vi "Fluidic Process.vi"(8 "error in":errorcluster) -> (0 "error out":errorcluster)   [LabVIEW 2019, in "Fluidic Process.lvlib"]
uses:
  Fluidic Process.lvlib
  User Event/Controls/UE Abort Action.ctl
  SubVI/Fluidic Para.ctl
  SubVI/Fluidic Data.ctl
  IO/sbRIO9623/SubVI/IO Control.ctl
  <vilib>/Utility/error.llb/Error Cluster From Error Code.vi
  <vilib>/ErrorRing/Error Ring.xnode
  Queues/Queues.lvlib
  Syringe Pump/NE-500/NE-500.lvlib
  Selection Valve/IDEX/IDEX.lvlib
  IO/sbRIO9623/sbRIO9623.lvlib
  LED/LED.lvlib
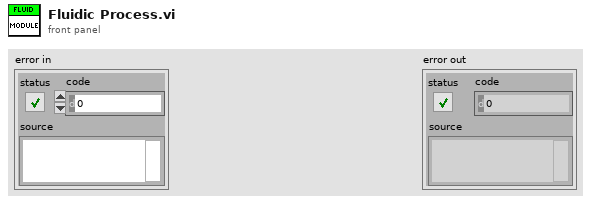
[diagram p1: front panel]
types:
  T1 = typedef "Fluidic Process.lvlib/Fluidic Para.ctl" = cluster{"Read Force Sensor":i32, "Read Regulator":i32, "Read Force Sensor?":bool, "Read Regulator?":bool, "Read Syringe Pump":i32, "Read Syringe Pump?":bool}
  T2 = typedef "Fluidic Process.lvlib/Fluidic Data.ctl" = cluster{"Step":i32, "Duration Time(s)":i32, "Syringe Pump Control":cluster{"Withdraw Rate (ul/min)":dbl, "Infuse Rate (ul/min)":dbl, "Direction":enum16{"Infuse", "Withdraw"}, "Syringe Diameter(mm)":dbl, "Syringe Pump Switch":bool}, "Selection Valve":enum16{"No Action", "Position 1", "Position 2", "Position 3", "Position 4", "Position 5", "Position 6"}, "Buffer Pinch Valve":cluster{"Buffer Load L":bool, "Buffer Load R":bool, "Buffer Chip L":bool, "Buffer Chip R":bool, "Sorting Waste":bool, "Filter Waste":bool, "Reagent Waste":bool, "Buffer Waste":bool, "Wash/Buffer Tank":bool}, "Blood Pinch Valve":cluster{"Load S1":bool, "Load S2":bool, "Blood in":bool}, "Regulator":cluster{"BL2 (V)":fxp<+,16,3>, "BL1 (V)":fxp<+,16,3>, "BR1 (V)":fxp<+,16,3>, "BR2 (V)":fxp<+,16,3>}, "Fast Valve":cluster{"Fast Valve 1":bool, "Fast Valve 2":bool}, "Air Valve":bool, "Blood Tube Latch1":bool, "Buffer Pump":bool, "Blood Sensor":cluster{"Calibrate Sensor 1":bool, "Calibrate Sensor 2":bool}, "Mirror Change":enum16{"Camera Side", "SiPM Side"}}
  T3 = cluster{"Fluidic Para":T1, "Total Process":i32, "Current Process":i32, "Tick Count":u32, "Duration(s)":dbl, "Fluidic Process":T2[], "Current Fluidic Process":T2, "Total Duration(s)":dbl, "Duration(s) Array":dbl[]}
  T4 = typedef "UE Abort Action.ctl" = enum16{"Create", "Get", "Destroy"}
  T5 = cluster{"Wdr Rate(UM)":dbl, "Inf Rate(UM)":dbl, "Dir":enum16{"Infuse", "Withdraw"}, "Dia(mm)":dbl}
  T6 = typedef "sbRIO9623.lvlib/IO Control.ctl" = cluster{"Regulator":cluster{"BL2 (V)":fxp<+,16,3>, "BL1 (V)":fxp<+,16,3>, "BR1 (V)":fxp<+,16,3>, "BR2 (V)":fxp<+,16,3>}, "Buffer Pinch Valve":cluster{"Buffer Load L":bool, "Buffer Load R":bool, "Buffer Chip L":bool, "Buffer Chip R":bool, "Sorting Waste":bool, "Filter Waste":bool, "Reagent Waste":bool, "Buffer Waste":bool, "Wash/Buffer Tank":bool}, "Blood Pinch Valve":cluster{"Load S1":bool, "Load S2":bool, "Blood in":bool}, "Fast Valve":cluster{"Fast Valve 1":bool, "Fast Valve 2":bool}, "Blood Sensor":cluster{"Calibrate Sensor 1":bool, "Calibrate Sensor 2":bool}, "Air Pressure":cluster{"Air Compressor":bool, "Air Compressor Manual":bool}, "Blood Tube Latch1":bool, "Air Valve":bool, "Buffer Pump":bool, "Mirror Change":enum16{"Camera Side", "SiPM Side"}}
  T7 = typedef "Fluidic Process.lvlib/SEQ Data.ctl" = cluster{"Fluidic Process Done?":bool, "Current Process":i32, "Remaining Time":dbl, "Total Process":i32, "Air Sealing":bool, "Force Condition":bool}
  T8 = typedef "LED.lvlib/SEQ Data.ctl" = cluster{"Initialize Sucess?":bool, "BL2 Regulator":dbl, "BL1 Regulator":dbl, "Blood Sensor 1":dbl, "Blood Sensor 2":dbl, "Air Pressure Sensor":dbl, "Force Snesor 1":u32, "Force Snesor 2":u32, "VI Refnum":refnum<vi>}
  T9 = cluster{"Withdraw Rate (ul/min)":dbl, "Infuse Rate (ul/min)":dbl, "Direction":enum16{"Infuse", "Withdraw"}, "Syringe Diameter(mm)":dbl, "Syringe Pump Switch":bool}
  T10 = enum16{"No Action", "Position 1", "Position 2", "Position 3", "Position 4", "Position 5", "Position 6"}
  T11 = typedef "NE-500.lvlib/SEQ Data.ctl" = cluster{"Status":string, "Initialize Done?":bool, "VI Refnum":refnum<vi>}
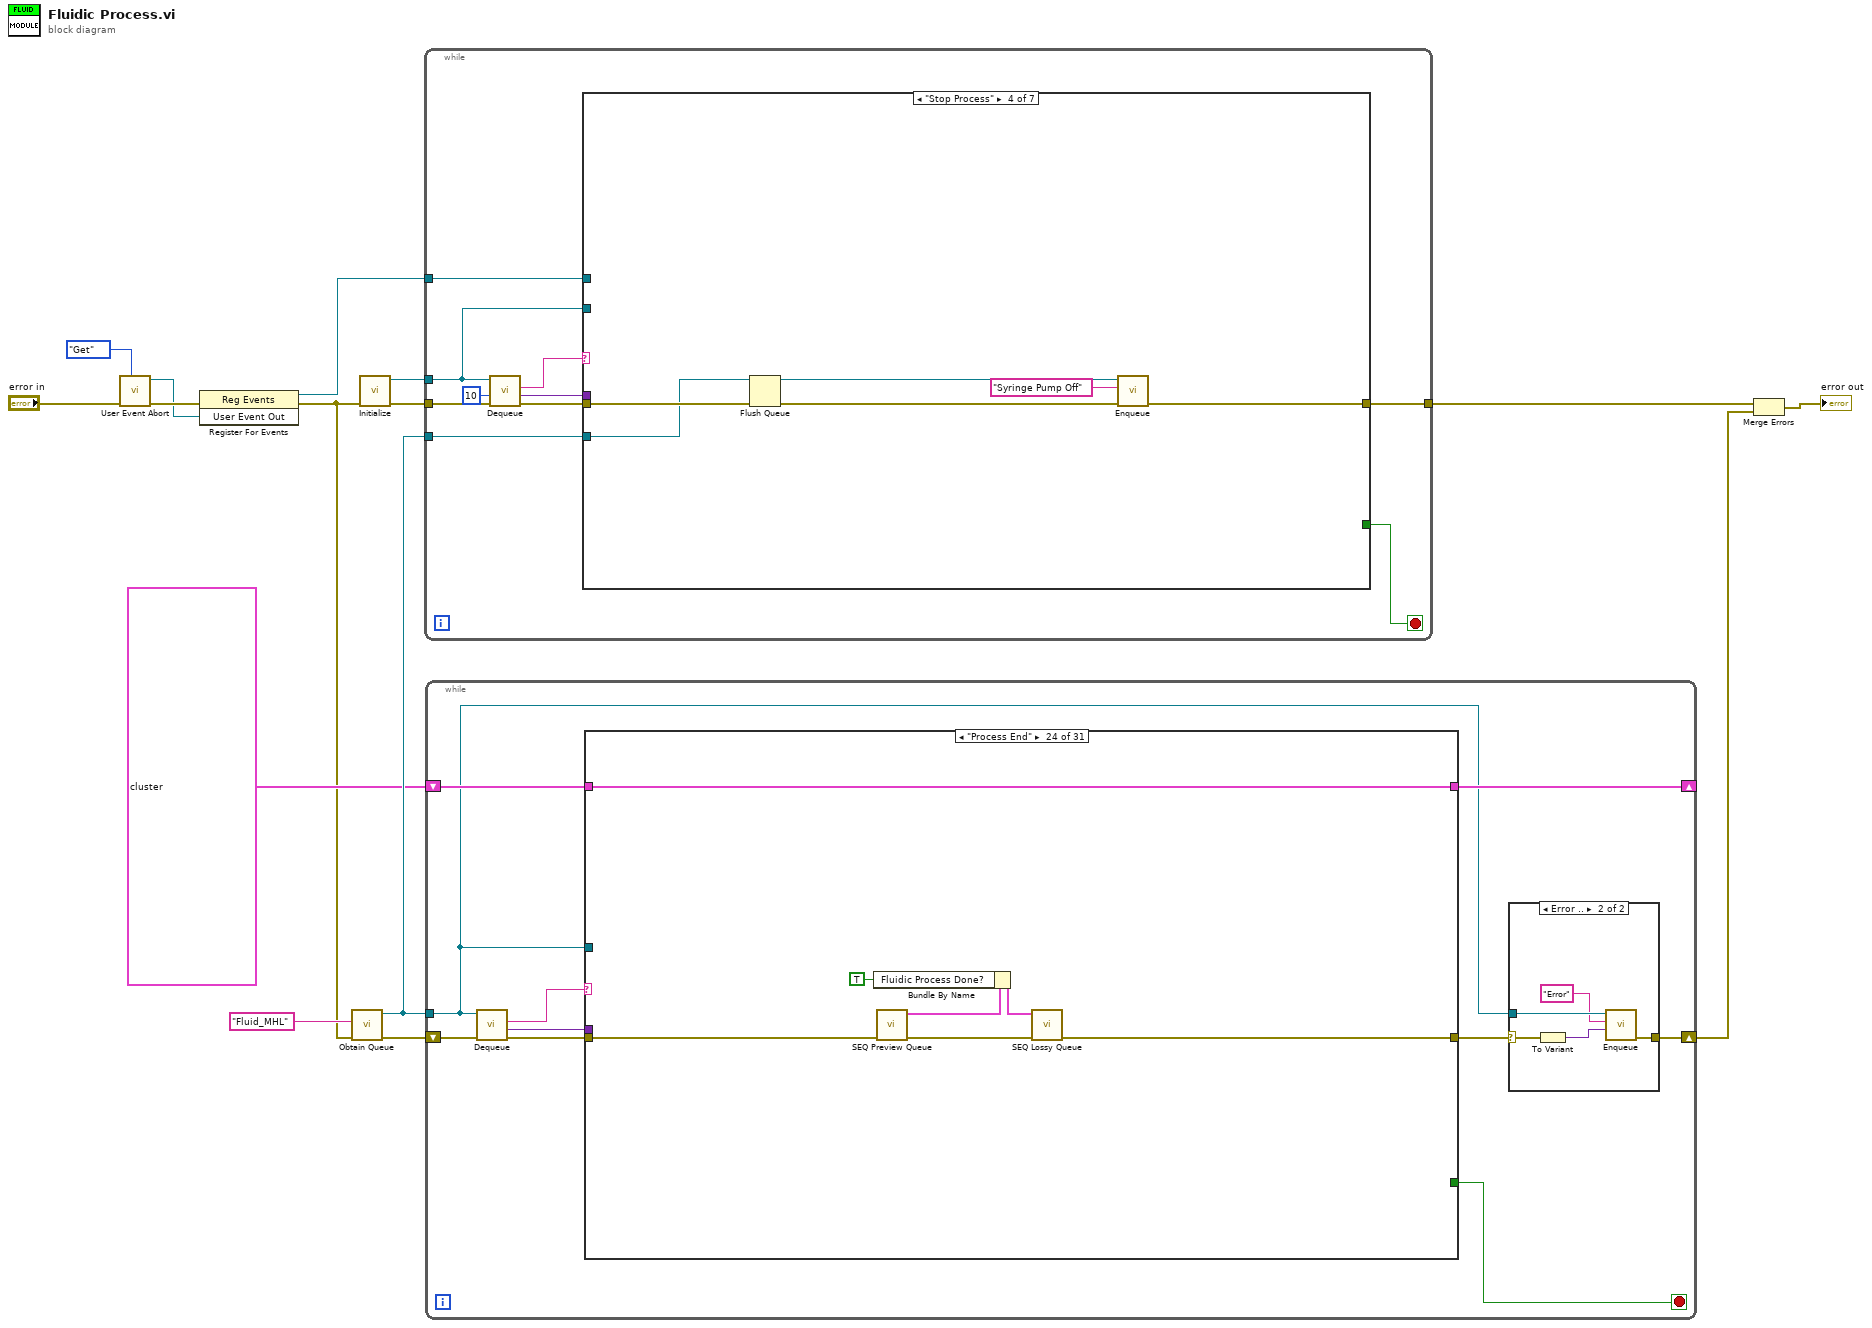
[diagram p0: block diagram]
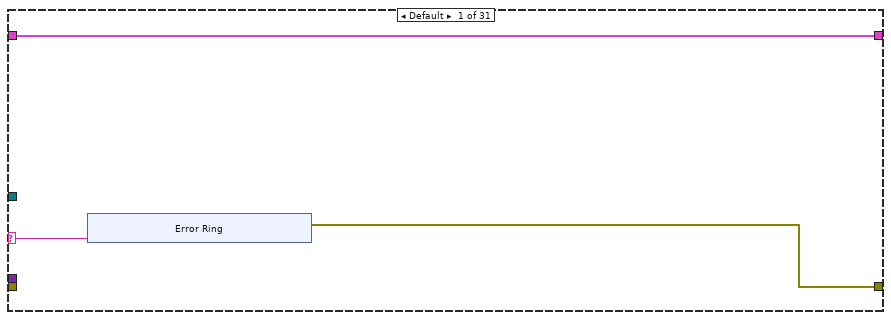
[diagram p2: hidden frame]
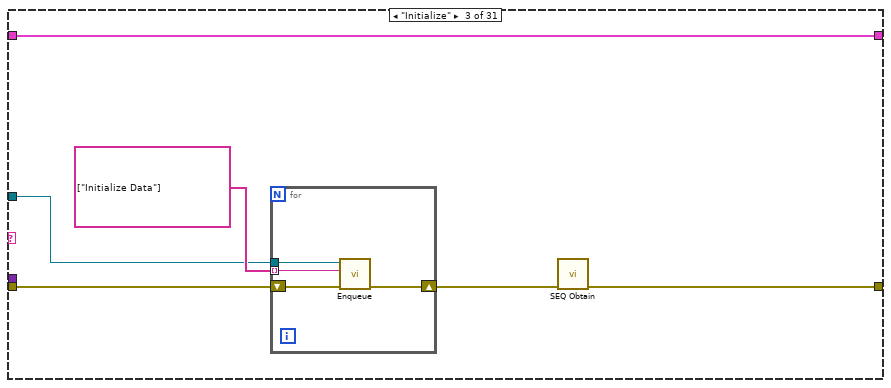
[diagram p4: hidden frame]
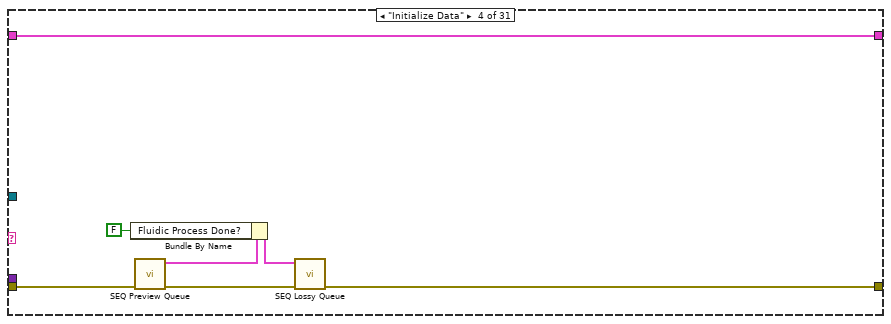
[diagram p5: hidden frame]
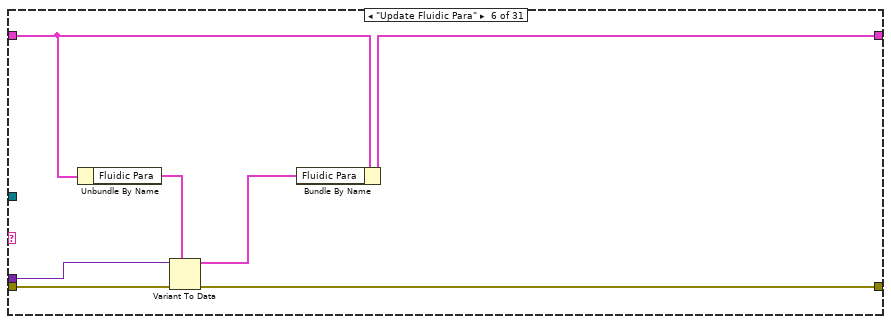
[diagram p7: hidden frame]
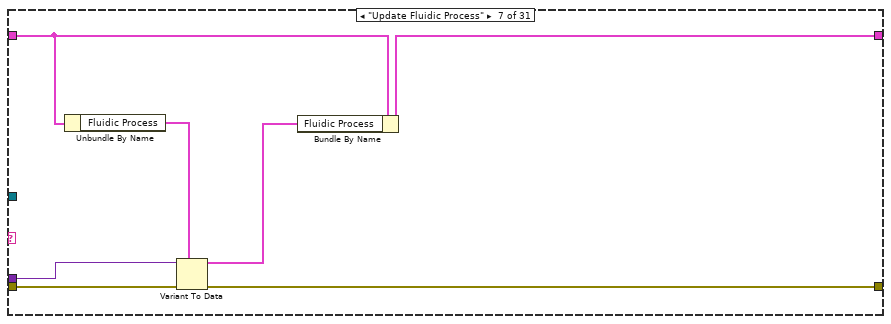
[diagram p8: hidden frame]
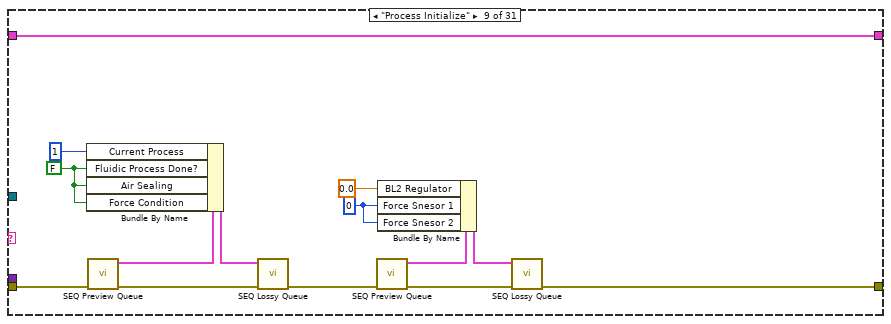
[diagram p10: hidden frame]
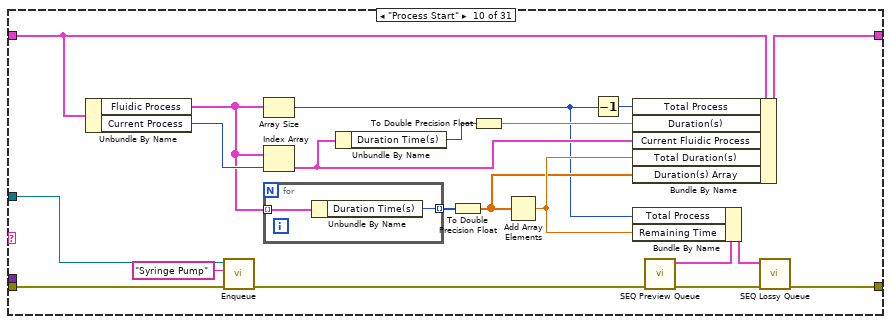
[diagram p11: hidden frame]
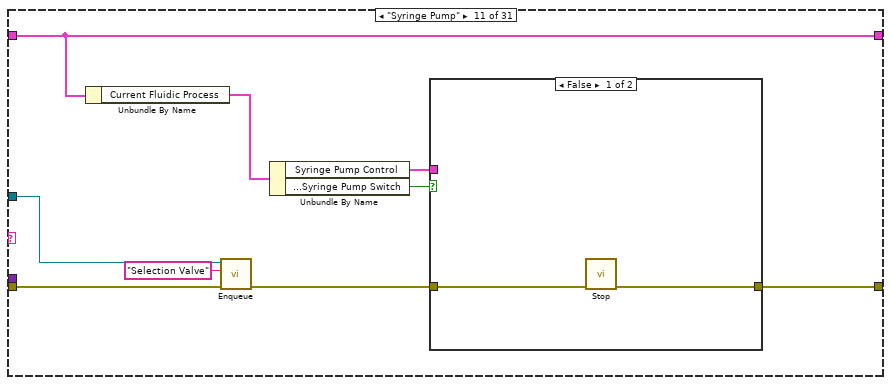
[diagram p12: hidden frame]
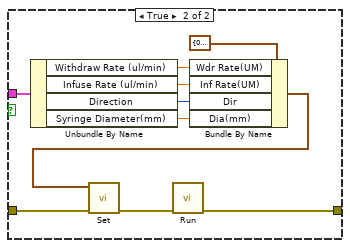
[diagram p13: hidden frame]
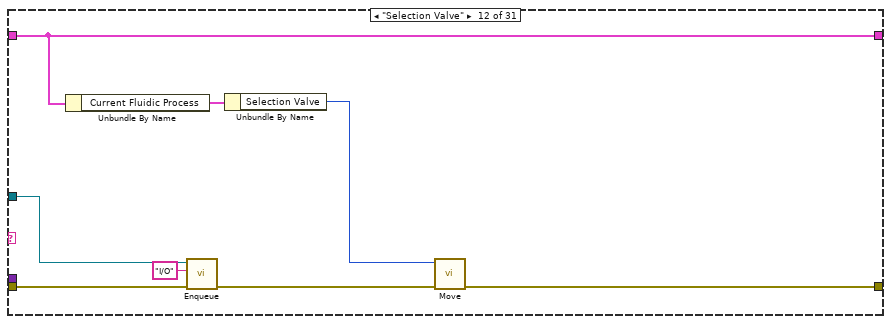
[diagram p14: hidden frame]
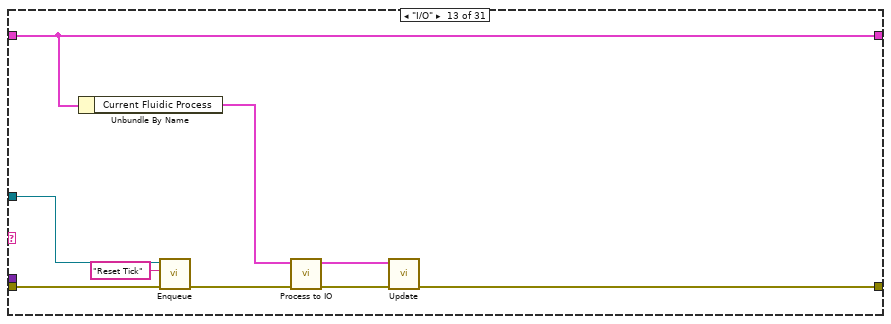
[diagram p15: hidden frame]
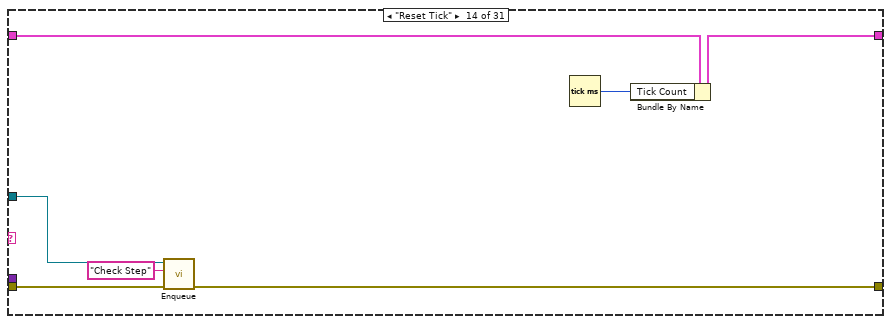
[diagram p16: hidden frame]
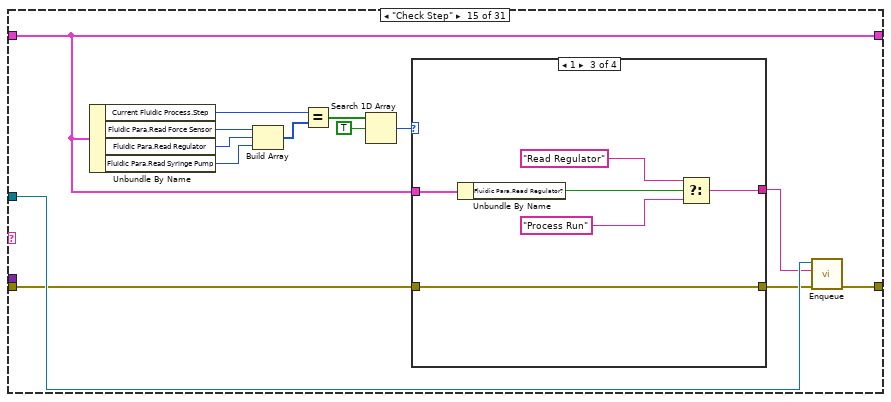
[diagram p17: hidden frame]
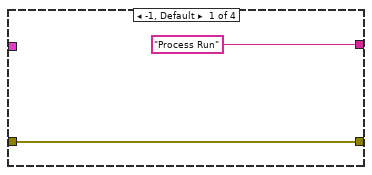
[diagram p18: hidden frame]
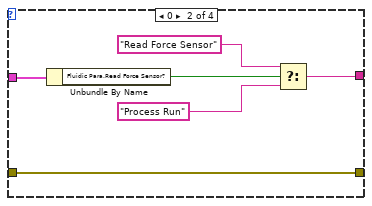
[diagram p19: hidden frame]
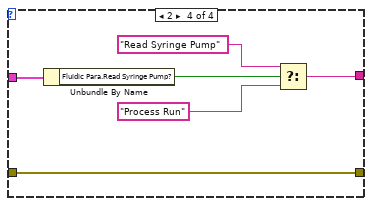
[diagram p20: hidden frame]
diagram:
  n1 = call "User Event Abort.vi"("Action"=UE_Abort_Action."Get", "Error In"="error in") -> ("Error Out"=w13:errorcluster, "User Event Out"=w12:refnum<user-event>)  [unwired: 8 in]
  n2 = register-events(error in=w13, w12) -> (reference out=w11:refnum<event-registration>, error out=w3:errorcluster)  [unwired: 1 in]
  n3 = call "Obtain Queue.vi"("Error In"=w3, "Queue Name"="Fluid_MHL") -> ("Error Out"=w9:errorcluster, "queue out"=w5:refnum<queue>)  [unwired: 8 in]
  n4 = call "Initialize.vi"("Error In"=w3) -> ("Error Out"=w2:errorcluster, "Queue out"=w1:refnum<queue>)  [unwired: 9 in]
  n5 = while {
    tunnel: w2 -> [w25]
    tunnel: w1 -> [w20]
    tunnel: [w19] -> w8
    tunnel: w11 -> [w18]
    tunnel: w5 -> [w16]
    stop <- w17 stop-if-true
    n6 = call "Dequeue.vi"("Error In"=w25, "timeout in ms (-1)"=10, "Queue in"=w20) -> ("Error Out"=w24:errorcluster, "Data"=w22:variant, "State"=w23:string)  [unwired: 5 in, 1 out]
    n7 = case shown="\"Stop Process\"" w23 {
      selector: w23 -> [w26 _ _ _ _ _ _]
      tunnel: w24 -> [w29 w33 w50 w60 w66 w70 w78]
      tunnel: w22 -> [_ _ w49 _ w63 _ _]
      tunnel: w20 -> [_ _ _ _ _ _ _]
      tunnel: [w29 w32 w43 w61 w65 w69 w77] -> w19
      tunnel: w18 -> [_ _ _ _ _ _ w76]
      tunnel: [_ _ _ _ _ TRUE _] -> w17
      tunnel: w16 -> [_ w31 w45 w58 w64 w68 _]
      frame "Typo", Default {
        n8 = Concatenate Strings("Typo: " ("string"), w26) -> (w28:string)
        n9 = One Button Dialog(message=w28) -> ()  [unwired: 1 in, 1 out]
      }
      frame "Initialize" {
        n10 = for {
          tunnel: w31 -> [w35]
          shift-right: [w36] -> w32
          shift-left: w33 -> [w37]
          tunnel: string[] ["Initialize"] -> [w34] mode=indexing
          n11 = call "Enqueue.vi"("Error In"=w37, "State"=w34, "Queue in"=w35) -> ("Error Out"=w36:errorcluster)  [unwired: 7 in, 1 out]
        }
      }
      frame "Run Process" {
        w40 = variant
        n12 = Variant To Data(error in=w50, type=string[][] [] ("Fluidic Process in"), Variant=w49) -> (data=w46:string[][], error out=w47:errorcluster)
        n13 = call "Prcoess Converter.vi"("error in"=w47, "Fluidic Process in"=w46) -> ("error out"=w44:errorcluster, "Fluidic Process out"=w42:T2[])  [unwired: 8 in]
        n14 = To Variant(anything=w42) -> (Variant=w41:variant)
        n15 = Build Array(w40, w41, w40) -> (w38:variant[])
        n16 = for {
          tunnel: w45 -> [w55]
          shift-right: [w53] -> w43
          shift-left: w44 -> [w54]
          tunnel: string[] ["Process Initialize", "Update Fluidic Process", "Process Start"] -> [w52] mode=indexing
          tunnel: w38 -> [w51] mode=indexing
          n17 = call "Enqueue.vi"("Error In"=w54, "Data"=w51, "State"=w52, "Queue in"=w55) -> ("Error Out"=w53:errorcluster)  [unwired: 6 in, 1 out]
        }
      }
      frame "Stop Process" {
        n18 = Flush Queue(queue=w58, error in (no error)=w60) -> (queue out=w57:refnum<queue>, error out=w59:errorcluster)  [unwired: 1 out]
        n19 = call "Enqueue.vi"("Error In"=w59, "State"="Syringe Pump Off", "Queue in"=w57) -> ("Error Out"=w61:errorcluster)  [unwired: 7 in, 1 out]
      }
      frame "Update Fluidic Para" {
        n20 = call "Enqueue.vi"("Error In"=w66, "Data"=w63, "State"="Update Fluidic Para", "Queue in"=w64) -> ("Error Out"=w65:errorcluster)  [unwired: 6 in, 1 out]
      }
      frame "Close" {
        n21 = for {
          tunnel: w68 -> [w73]
          shift-right: [w74] -> w69
          shift-left: w70 -> [w75]
          tunnel: string[] ["Close"] -> [w72] mode=indexing
          n22 = call "Enqueue.vi"("Error In"=w75, "State"=w72, "Queue in"=w73) -> ("Error Out"=w74:errorcluster)  [unwired: 7 in, 1 out]
        }
      }
      frame "Idle" {
        n23 = event shown="[1] <User Event Out>: User Event" {
          selector: w76 -> [_ w84]
          dyn-events: _ -> [_ _]
          timeout: 10 -> [_ _]
          tunnel: w78 -> [w80 w82]
          tunnel: [w80 w83] -> w77
          event Timeout {
            n24 = event-data() -> ()  [unwired: 1 in, 3 out]
          }
          event User Event {
            n25 = event-data() -> ()  [unwired: 1 in, 4 out]
            n26 = call "Close.vi"("Error In"=w82) -> ("Error Out"=w81:errorcluster)  [unwired: 10 in]
            n27 = Unregister For Events(event registration refnum=w84, error in=w81) -> (error out=w83:errorcluster)
          }
        }
      }
    }
  }
  n28 = while {
    tunnel: w5 -> [w86]
    shift-right: [w89] -> _
    shift-left: T3 {"Fluidic Para"={"Read Force Sensor"=0, "Read Regulator"=0, "Read Force Sensor?"=FALSE, "Read Regulator?"=FALSE, "Read Syringe Pump"=0, "Read Syringe Pump?"=FALSE}, "Total Process"=0, "Current Process"=0, "Tick Count"=0, "Duration(s)"=0.0, "Fluidic Process"=[], "Current Fluidic Process"={"Step"=0, "Duration Time(s)"=0, "Syringe Pump Control"={"Withdraw Rate (ul/min)"=0.0, "Infuse Rate (ul/min)"=0.0, "Direction"=enum."Infuse", "Syringe Diameter(mm)"=0.0, "Syringe Pump Switch"=FALSE}, "Selection Valve"=enum."No Action", "Buffer Pinch Valve"={"Buffer Load L"=FALSE, "Buffer Load R"=FALSE, "Buffer Chip L"=FALSE, "Buffer Chip R"=FALSE, "Sorting Waste"=FALSE, "Filter Waste"=FALSE, "Reagent Waste"=FALSE, "Buffer Waste"=FALSE, "Wash/Buffer Tank"=FALSE}, "Blood Pinch Valve"={"Load S1"=FALSE, "Load S2"=FALSE, "Blood in"=FALSE}, "Regulator"={"BL2 (V)"=0.0, "BL1 (V)"=0.0, "BR1 (V)"=0.0, "BR2 (V)"=0.0}, "Fast Valve"={"Fast Valve 1"=FALSE, "Fast Valve 2"=FALSE}, "Air Valve"=FALSE, "Blood Tube Latch1"=FALSE, "Buffer Pump"=FALSE, "Blood Sensor"={"Calibrate Sensor 1"=FALSE, "Calibrate Sensor 2"=FALSE}, "Mirror Change"=enum."Camera Side"}, "Total Duration(s)"=0.0, "Duration(s) Array"=[]} -> [w90]
    shift-right: [w88] -> w6
    shift-left: w9 -> [w94]
    stop <- w85 stop-if-true
    n29 = call "Dequeue.vi"("Error In"=w94, "Queue in"=w86) -> ("Error Out"=w91:errorcluster, "Data"=w92:variant, "State"=w93:string)  [unwired: 6 in, 1 out]
    n30 = case shown="\"Process End\"" w93 {
      selector: w93 -> [w96 _ _ _ _ _ _ _ _ _ _ _ _ _ _ _ _ _ _ _ _ _ _ _ _ _ _ _ _ _ _]
      tunnel: w86 -> [_ _ w110 _ _ _ _ _ _ w170 w185 w205 w214 w220 w235 w260 w266 w271 w297 w334 w369 w404 w417 _ w455 w464 _ _ _ w479 w489]
      tunnel: w92 -> [_ _ _ _ _ w131 w138 _ _ _ _ _ _ _ _ _ _ _ _ _ _ _ _ _ _ _ _ w471 _ _ _]
      tunnel: w91 -> [_ w105 w111 w122 w125 w132 w139 w140 w155 w173 w186 w206 w215 w221 w225 w261 w267 w272 w298 w324 w359 w379 w419 w449 w456 w465 w468 w472 w476 w480 w490]
      tunnel: w90 -> [w97 w106 w109 w123 w124 w130 w137 w141 w142 w175 w184 w204 w213 w222 w226 w262 w268 w273 w279 w315 w348 w393 w426 w450 w457 w466 w467 w469 w475 w477 w488]
      tunnel: [w97 w106 w109 w123 w124 w128 w135 w141 w142 w174 w184 w204 w213 w217 w226 w262 w268 w273 w279 w315 w348 w393 w425 w450 w457 w466 w467 w469 w475 w477 w488] -> w89
      tunnel: [w95 w105 w107 w120 w125 w126 w133 w140 w148 w162 w180 w200 w208 w218 w236 w258 w264 w269 w284 w311 w353 w389 w413 w447 w451 w461 w468 errorcluster {"status"=FALSE, "code"=0, "source"=""} ("Error Out") w476 w478 w486] -> w87
      tunnel: [_ _ _ _ _ _ _ _ _ _ _ _ _ _ _ _ _ _ _ _ _ _ _ _ _ _ _ _ _ _ TRUE] -> w85
      frame Default {
        n31 = xnode "Error Ring"("parameter 0"=w96) -> ("error out"=w95:errorcluster)
      }
      frame "------Initialize------" {
      }
      frame "Initialize" {
        n32 = for {
          tunnel: w110 -> [w114]
          shift-right: [w115] -> w108
          shift-left: w111 -> [w116]
          tunnel: string[] ["Initialize Data"] -> [w113] mode=indexing
          n33 = call "Enqueue.vi"("Error In"=w116, "State"=w113, "Queue in"=w114) -> ("Error Out"=w115:errorcluster)  [unwired: 7 in, 1 out]
        }
        n34 = call "SEQ Obtain.vi"("error in"=w108) -> ("error out"=w107:errorcluster)  [unwired: 9 in, 1 out]
      }
      frame "Initialize Data" {
        n35 = call "SEQ Preview Queue.vi"("error in"=w122) -> ("error out"=w121:errorcluster, "SEQ Data"=w119:T7)  [unwired: 9 in]
        n36 = Bundle By Name(cluster=w119, "Fluidic Process Done?"=FALSE) -> (w118:T7)
        n37 = call "SEQ Lossy Queue.vi"("error in"=w121, "SEQ Data"=w118) -> ("error out"=w120:errorcluster)  [unwired: 9 in]
      }
      frame "------Functions------" {
      }
      frame "Update Fluidic Para" {
        n38 = Unbundle By Name(w130) -> ("Fluidic Para"=w129:T1)
        n39 = Variant To Data(error in=w132, type=w129, Variant=w131) -> (data=w127:T1, error out=w126:errorcluster)
        n40 = Bundle By Name(cluster=w130, "Fluidic Para"=w127) -> (w128:T3)
      }
      frame "Update Fluidic Process" {
        n41 = Unbundle By Name(w137) -> ("Fluidic Process"=w136:T2[])
        n42 = Variant To Data(error in=w139, type=w136, Variant=w138) -> (data=w134:T2[], error out=w133:errorcluster)
        n43 = Bundle By Name(cluster=w137, "Fluidic Process"=w134) -> (w135:T3)
      }
      frame "------Process------" {
      }
      frame "Process Initialize" {
        w144 = u32 0 ("Force Snesor 1")
        w143 = FALSE ("Fluidic Process Done?")
        n44 = call "SEQ Preview Queue.vi"("error in"=w155) -> ("error out"=w154:errorcluster, "SEQ Data"=w153:T7)  [unwired: 9 in]
        n45 = Bundle By Name(cluster=w153, "Current Process"=1, "Fluidic Process Done?"=w143, "Air Sealing"=w143, "Force Condition"=w143) -> (w152:T7)
        n46 = call "SEQ Lossy Queue.vi"("error in"=w154, "SEQ Data"=w152) -> ("error out"=w150:errorcluster)  [unwired: 9 in]
        n47 = call "SEQ Preview Queue.vi"("error in"=w150) -> ("error out"=w149:errorcluster, "SEQ Data"=w147:T8)  [unwired: 9 in]
        n48 = Bundle By Name(cluster=w147, "BL2 Regulator"=0.0, "Force Snesor 1"=w144, "Force Snesor 2"=w144) -> (w146:T8)
        n49 = call "SEQ Lossy Queue.vi"("error in"=w149, "SEQ Data"=w146) -> ("error out"=w148:errorcluster)  [unwired: 9 in]
      }
      frame "Process Start" {
        n50 = Unbundle By Name(w175) -> ("Fluidic Process"=w165:T2[], "Current Process"=w171:i32)
        n51 = call "Enqueue.vi"("Error In"=w173, "State"="Syringe Pump", "Queue in"=w170) -> ("Error Out"=w164:errorcluster)  [unwired: 7 in, 1 out]
        n52 = Array Size(array=w165) -> (size(s)=w156:i32)
        n53 = Index Array(array=w165, index=w171) -> (element=w168:T2)
        n54 = for {
          tunnel: w165 -> [w177] mode=indexing
          tunnel: [w176] -> w159 mode=indexing
          n55 = Unbundle By Name(w177) -> ("Duration Time(s)"=w176:i32)
        }
        n56 = Unbundle By Name(w168) -> ("Duration Time(s)"=w167:i32)
        n57 = To Double Precision Float(number=w159) -> (double precision float=w157:dbl[])
        n58 = To Double Precision Float(number=w167) -> (double precision float=w166:dbl)
        n59 = Add Array Elements(numeric array=w157) -> (sum=w158:dbl)
        n60 = Decrement(x=w156) -> (x-1=w172:i32)
        n61 = Bundle By Name(cluster=w175, "Total Process"=w172, "Duration(s)"=w166, "Current Fluidic Process"=w168, "Total Duration(s)"=w158, "Duration(s) Array"=w157) -> (w174:T3)
        n62 = call "SEQ Preview Queue.vi"("error in"=w164) -> ("error out"=w163:errorcluster, "SEQ Data"=w161:T7)  [unwired: 9 in]
        n63 = Bundle By Name(cluster=w161, "Total Process"=w156, "Remaining Time"=w158) -> (w160:T7)
        n64 = call "SEQ Lossy Queue.vi"("error in"=w163, "SEQ Data"=w160) -> ("error out"=w162:errorcluster)  [unwired: 9 in]
      }
      frame "Syringe Pump" {
        n65 = Unbundle By Name(w184) -> ("Current Fluidic Process"=w183:T2)
        n66 = call "Enqueue.vi"("Error In"=w186, "State"="Selection Valve", "Queue in"=w185) -> ("Error Out"=w181:errorcluster)  [unwired: 7 in, 1 out]
        n67 = Unbundle By Name(w183) -> ("Syringe Pump Control"=w179:T9, "Syringe Pump Control.Syringe Pump Switch"=w182:bool)
        n68 = case shown="False" w182 {
          tunnel: w181 -> [w188 w198]
          tunnel: [w187 w189] -> w180
          tunnel: w179 -> [_ w196]
          frame False {
            n69 = call "Stop.vi"("Error In"=w188) -> ("Error Out"=w187:errorcluster)  [unwired: 10 in]
          }
          frame True {
            n70 = Unbundle By Name(w196) -> ("Withdraw Rate (ul/min)"=w194:dbl, "Infuse Rate (ul/min)"=w193:dbl, "Direction"=w192:enum16{"Infuse", "Withdraw"}, "Syringe Diameter(mm)"=w191:dbl)
            n71 = Bundle By Name(cluster=T5 {"Wdr Rate(UM)"=0.0, "Inf Rate(UM)"=0.0, "Dir"=enum."Infuse", "Dia(mm)"=0.0} ("Setting"), "Wdr Rate(UM)"=w194, "Inf Rate(UM)"=w193, "Dir"=w192, "Dia(mm)"=w191) -> (w190:T5)
            n72 = call "Set.vi"("Error In"=w198, "Setting"=w190) -> ("Error Out"=w197:errorcluster)  [unwired: 9 in]
            n73 = call "Run.vi"("Error In"=w197) -> ("Error Out"=w189:errorcluster)  [unwired: 10 in]
          }
        }
      }
      frame "Selection Valve" {
        n74 = Unbundle By Name(w204) -> ("Current Fluidic Process"=w203:T2)
        n75 = call "Enqueue.vi"("Error In"=w206, "State"="I/O", "Queue in"=w205) -> ("Error Out"=w201:errorcluster)  [unwired: 7 in, 1 out]
        n76 = Unbundle By Name(w203) -> ("Selection Valve"=w202:T10)
        n77 = call "Move.vi"("Error In"=w201, "Position"=w202) -> ("Error Out"=w200:errorcluster)  [unwired: 9 in]
      }
      frame "I/O" {
        n78 = Unbundle By Name(w213) -> ("Current Fluidic Process"=w212:T2)
        n79 = call "Enqueue.vi"("Error In"=w215, "State"="Reset Tick", "Queue in"=w214) -> ("Error Out"=w211:errorcluster)  [unwired: 7 in, 1 out]
        n80 = call "Process to IO.vi"("error in"=w211, "Process in"=w212) -> ("error out"=w210:errorcluster, "Process out"=w209:T6)  [unwired: 8 in]
        n81 = call "Update.vi"("Error In"=w210, "I/O Control"=w209) -> ("Error Out"=w208:errorcluster)  [unwired: 9 in]
      }
      frame "Reset Tick" {
        n82 = call "Enqueue.vi"("Error In"=w221, "State"="Check Step", "Queue in"=w220) -> ("Error Out"=w218:errorcluster)  [unwired: 7 in, 1 out]
        n83 = Tick Count (ms)() -> (millisecond timer value=w216:u32)
        n84 = Bundle By Name(cluster=w222, "Tick Count"=w216) -> (w217:T3)
      }
      frame "Check Step" {
        n85 = Unbundle By Name(w226) -> ("Current Fluidic Process.Step"=w231:i32, "Fluidic Para.Read Force Sensor"=w234:i32, "Fluidic Para.Read Regulator"=w233:i32, "Fluidic Para.Read Syringe Pump"=w232:i32)
        n86 = Build Array(w234, w233, w232) -> (w230:i32[])
        n87 = Equal?(x=w231, y=w230) -> (x = y?=w229:bool[])
        n88 = Search 1D Array(1D array=w229, element=TRUE) -> (index of element=w227:i32)  [unwired: 1 in]
        n89 = case shown="1" w227 {
          tunnel: w226 -> [_ w243 w249 w255]
          tunnel: w225 -> [w238 w244 w250 w256]
          tunnel: [w238 w244 w250 w256] -> w224
          tunnel: ["Process Run" w239 w245 w251] -> w223
          frame -1, Default {
          }
          frame 0 {
            n90 = Unbundle By Name(w243) -> ("Fluidic Para.Read Force Sensor?"=w240:bool)
            n91 = Select(t="Read Force Sensor", s=w240, f="Process Run") -> (s? t:f=w239:string)
          }
          frame 1 {
            n92 = Unbundle By Name(w249) -> ("Fluidic Para.Read Regulator?"=w246:bool)
            n93 = Select(t="Read Regulator", s=w246, f="Process Run") -> (s? t:f=w245:string)
          }
          frame 2 {
            n94 = Unbundle By Name(w255) -> ("Fluidic Para.Read Syringe Pump?"=w252:bool)
            n95 = Select(t="Read Syringe Pump", s=w252, f="Process Run") -> (s? t:f=w251:string)
          }
        }
        n96 = call "Enqueue.vi"("Error In"=w224, "State"=w223, "Queue in"=w235) -> ("Error Out"=w236:errorcluster)  [unwired: 7 in, 1 out]
      }
      frame "Read Force Sensor" {
        n97 = call "Enqueue.vi"("Error In"=w261, "State"="Process Run_Force Sensor", "Queue in"=w260) -> ("Error Out"=w259:errorcluster)  [unwired: 7 in, 1 out]
        n98 = call "Read Force Sensor.vi"("Error In"=w259) -> ("Error Out"=w258:errorcluster)  [unwired: 10 in]
      }
      frame "Read Regulator" {
        n99 = call "Enqueue.vi"("Error In"=w267, "State"="Process Run_Regulator", "Queue in"=w266) -> ("Error Out"=w265:errorcluster)  [unwired: 7 in, 1 out]
        n100 = call "Read BL2 Regulator.vi"("Error In"=w265) -> ("Error Out"=w264:errorcluster)  [unwired: 10 in]
      }
      frame "Read Syringe Pump" {
        n101 = call "Enqueue.vi"("Error In"=w272, "State"="Process Run_Syringe Pump", "Queue in"=w271) -> ("Error Out"=w269:errorcluster)  [unwired: 7 in, 1 out]
      }
      frame "Process Run" {
        n102 = Unbundle By Name(w279) -> ("Total Duration(s)"=w281:dbl, "Tick Count"=w296:u32, "Duration(s)"=w291:dbl)
        n103 = Tick Count (ms)() -> (millisecond timer value=w295:u32)
        n104 = Subtract(x=w295, y=w296) -> (x-y=w294:u32)
        n105 = To Double Precision Float(number=w294) -> (double precision float=w293:dbl)
        n106 = Divide(x=w293, y=1000.0) -> (x/y=w280:dbl)
        n107 = Wait (ms)(milliseconds to wait=u32 100) -> ()  [unwired: 1 out]
        n108 = Greater Or Equal?(x=w280, y=w291) -> (x >= y?=w290:bool)
        n109 = Subtract(x=w281, y=w280) -> (x-y=w274:dbl)
        n110 = Select(t="Process Next", s=w290, f="Process Run") -> (s? t:f=w287:string)
        n111 = Less?(x=w274, y=0.0) -> (x < y?=w276:bool)
        n112 = Select(t=0.0, s=w276, f=w274) -> (s? t:f=w277:dbl)
        n113 = call "Enqueue.vi"("Error In"=w298, "State"=w287, "Queue in"=w297) -> ("Error Out"=w286:errorcluster)  [unwired: 7 in, 1 out]
        n114 = call "SEQ Preview Queue.vi"("error in"=w286) -> ("error out"=w285:errorcluster, "SEQ Data"=w283:T7)  [unwired: 9 in]
        n115 = Bundle By Name(cluster=w283, "Remaining Time"=w277) -> (w282:T7)
        n116 = call "SEQ Lossy Queue.vi"("error in"=w285, "SEQ Data"=w282) -> ("error out"=w284:errorcluster)  [unwired: 9 in]
      }
      frame "Process Run_Force Sensor" {
        w319 = u32 220 ("y")
        n117 = Unbundle By Name(w315) -> ("Total Duration(s)"=w314:dbl, "Tick Count"=w333:u32, "Duration(s)"=w328:dbl)
        n118 = call "SEQ Preview Queue.vi"("error in"=w324) -> ("error out"=w323:errorcluster, "SEQ Data"=w322:T8)  [unwired: 9 in]
        n119 = Unbundle By Name(w322) -> ("Force Snesor 1"=w321:u32, "Force Snesor 2"=w320:u32)
        n120 = Tick Count (ms)() -> (millisecond timer value=w332:u32)
        n121 = Subtract(x=w332, y=w333) -> (x-y=w331:u32)
        n122 = To Double Precision Float(number=w331) -> (double precision float=w330:dbl)
        n123 = Greater Or Equal?(x=w321, y=w319) -> (x >= y?=w318:bool)
        n124 = Greater Or Equal?(x=w320, y=w319) -> (x >= y?=w317:bool)
        n125 = Divide(x=w330, y=1000.0) -> (x/y=w313:dbl)
        n126 = Greater Or Equal?(x=w313, y=w328) -> (x >= y?=w316:bool)
        n127 = And(x=w318, y=w317) -> (x .and. y?=w300:bool)
        n128 = Wait (ms)(milliseconds to wait=u32 100) -> ()  [unwired: 1 out]
        n129 = Or(x=w316, y=w300) -> (x .or. y?=w301:bool)
        n130 = Subtract(x=w314, y=w313) -> (x-y=w305:dbl)
        n131 = Select(t="Process Next", s=w301, f="Process Run_Force Sensor") -> (s? t:f=w325:string)
        n132 = Less?(x=w305, y=0.0) -> (x < y?=w307:bool)
        n133 = call "Enqueue.vi"("Error In"=w323, "State"=w325, "Queue in"=w334) -> ("Error Out"=w303:errorcluster)  [unwired: 7 in, 1 out]
        n134 = Select(t=0.0, s=w307, f=w305) -> (s? t:f=w304:dbl)
        n135 = case shown="True" w301 {
          tunnel: w303 -> [w336 w338]
          tunnel: [w336 w337] -> w302
          frame False {
          }
          frame True {
            n136 = call "Stop Read.vi"("Error In"=w338) -> ("Error Out"=w337:errorcluster)  [unwired: 10 in]
          }
        }
        n137 = call "SEQ Preview Queue.vi"("error in"=w302) -> ("error out"=w312:errorcluster, "SEQ Data"=w310:T7)  [unwired: 9 in]
        n138 = Bundle By Name(cluster=w310, "Remaining Time"=w304, "Force Condition"=w300) -> (w309:T7)
        n139 = call "SEQ Lossy Queue.vi"("error in"=w312, "SEQ Data"=w309) -> ("error out"=w311:errorcluster)  [unwired: 9 in]
      }
      frame "Process Run_Regulator" {
        n140 = Unbundle By Name(w348) -> ("Total Duration(s)"=w350:dbl, "Tick Count"=w368:u32, "Duration(s)"=w363:dbl)
        n141 = call "SEQ Preview Queue.vi"("error in"=w359) -> ("error out"=w358:errorcluster, "SEQ Data"=w357:T8)  [unwired: 9 in]
        n142 = Unbundle By Name(w357) -> ("BL2 Regulator"=w356:dbl)
        n143 = Tick Count (ms)() -> (millisecond timer value=w367:u32)
        n144 = Subtract(x=w367, y=w368) -> (x-y=w366:u32)
        n145 = To Double Precision Float(number=w366) -> (double precision float=w365:dbl)
        n146 = Greater?(x=w356, y=4.5) -> (0:w340:bool)
        n147 = Divide(x=w365, y=1000.0) -> (x/y=w349:dbl)
        n148 = Subtract(x=w350, y=w349) -> (x-y=w344:dbl)
        n149 = Greater Or Equal?(x=w349, y=w363) -> (x >= y?=w339:bool)
        n150 = Wait (ms)(milliseconds to wait=u32 100) -> ()  [unwired: 1 out]
        n151 = Select(t="Process Next", s=w339, f="Process Run_Regulator") -> (s? t:f=w360:string)
        n152 = Less?(x=w344, y=0.0) -> (x < y?=w346:bool)
        n153 = call "Enqueue.vi"("Error In"=w358, "State"=w360, "Queue in"=w369) -> ("Error Out"=w342:errorcluster)  [unwired: 7 in, 1 out]
        n154 = Select(t=0.0, s=w346, f=w344) -> (s? t:f=w343:dbl)
        n155 = case shown="False" w339 {
          tunnel: w342 -> [w371 w373]
          tunnel: [w371 w372] -> w341
          frame False {
          }
          frame True {
            n156 = call "Stop Read.vi"("Error In"=w373) -> ("Error Out"=w372:errorcluster)  [unwired: 10 in]
          }
        }
        n157 = call "SEQ Preview Queue.vi"("error in"=w341) -> ("error out"=w354:errorcluster, "SEQ Data"=w352:T7)  [unwired: 9 in]
        n158 = Bundle By Name(cluster=w352, "Remaining Time"=w343, "Air Sealing"=w340) -> (w351:T7)
        n159 = call "SEQ Lossy Queue.vi"("error in"=w354, "SEQ Data"=w351) -> ("error out"=w353:errorcluster)  [unwired: 9 in]
      }
      frame "Process Run_Syringe Pump" {
        n160 = Unbundle By Name(w393) -> ("Total Duration(s)"=w392:dbl, "Tick Count"=w403:u32, "Duration(s)"=w398:dbl)
        n161 = call "SEQ Preview Queue.vi"("error in"=w379) -> ("error out"=w378:errorcluster, "SEQ Data"=w377:T11)  [unwired: 9 in]
        n162 = Unbundle By Name(w377) -> ("Status"=w376:string)
        n163 = Tick Count (ms)() -> (millisecond timer value=w402:u32)
        n164 = Subtract(x=w402, y=w403) -> (x-y=w401:u32)
        n165 = Equal?(x=w376, y="P") -> (x = y?=w374:bool)
        n166 = To Double Precision Float(number=w401) -> (double precision float=w400:dbl)
        n167 = Divide(x=w400, y=1000.0) -> (x/y=w391:dbl)
        n168 = Greater Or Equal?(x=w391, y=w398) -> (x >= y?=w394:bool)
        n169 = Wait (ms)(milliseconds to wait=u32 100) -> ()  [unwired: 1 out]
        n170 = Or(x=w394, y=w374) -> (x .or. y?=w380:bool)
        n171 = Subtract(x=w392, y=w391) -> (x-y=w383:dbl)
        n172 = Select(t="Process Next", s=w380, f="Process Run_Syringe Pump") -> (s? t:f=w395:string)
        n173 = Less?(x=w383, y=0.0) -> (x < y?=w385:bool)
        n174 = call "Enqueue.vi"("Error In"=w378, "State"=w395, "Queue in"=w404) -> ("Error Out"=w381:errorcluster)  [unwired: 7 in, 1 out]
        n175 = Select(t=0.0, s=w385, f=w383) -> (s? t:f=w382:dbl)
        n176 = call "SEQ Preview Queue.vi"("error in"=w381) -> ("error out"=w390:errorcluster, "SEQ Data"=w388:T7)  [unwired: 9 in]
        n177 = Bundle By Name(cluster=w388, "Remaining Time"=w382) -> (w387:T7)
        n178 = call "SEQ Lossy Queue.vi"("error in"=w390, "SEQ Data"=w387) -> ("error out"=w389:errorcluster)  [unwired: 9 in]
      }
      frame "Process Next" {
        n179 = Unbundle By Name(w426) -> ("Total Process"=w424:i32, "Current Process"=w422:i32, "Fluidic Process"=w421:T2[], "Duration(s) Array"=w409:dbl[])
        n180 = Equal?(x=w424, y=w422) -> (x = y?=w423:bool)
        n181 = case shown="False" w423 {
          tunnel: w419 -> [w437 w443]
          tunnel: [w437 w443] -> w418
          tunnel: w422 -> [w434 _]
          tunnel: w421 -> [w435 _]
          tunnel: [w431 0] -> w410
          tunnel: [w428 T2 {"Step"=0, "Duration Time(s)"=0, "Syringe Pump Control"={"Withdraw Rate (ul/min)"=0.0, "Infuse Rate (ul/min)"=0.0, "Direction"=enum."Infuse", "Syringe Diameter(mm)"=0.0, "Syringe Pump Switch"=FALSE}, "Selection Valve"=enum."No Action", "Buffer Pinch Valve"={"Buffer Load L"=FALSE, "Buffer Load R"=FALSE, "Buffer Chip L"=FALSE, "Buffer Chip R"=FALSE, "Sorting Waste"=FALSE, "Filter Waste"=FALSE, "Reagent Waste"=FALSE, "Buffer Waste"=FALSE, "Wash/Buffer Tank"=FALSE}, "Blood Pinch Valve"={"Load S1"=FALSE, "Load S2"=FALSE, "Blood in"=FALSE}, "Regulator"={"BL2 (V)"=0.0, "BL1 (V)"=0.0, "BR1 (V)"=0.0, "BR2 (V)"=0.0}, "Fast Valve"={"Fast Valve 1"=FALSE, "Fast Valve 2"=FALSE}, "Air Valve"=FALSE, "Blood Tube Latch1"=FALSE, "Buffer Pump"=FALSE, "Blood Sensor"={"Calibrate Sensor 1"=FALSE, "Calibrate Sensor 2"=FALSE}, "Mirror Change"=enum."Camera Side"} ("Cluster")] -> w420
          tunnel: ["Syringe Pump" "Process End"] -> w416
          tunnel: w409 -> [w432 _]
          tunnel: [w433 w439] -> w408
          tunnel: [w429 w439] -> w407
          tunnel: [w427 1 ("Step")] -> w406
          frame False {
            n182 = Increment(x=w434) -> (x+1=w431:i32)
            n183 = Index Array(array=w435, index=w431) -> (element=w428:T2)
            n184 = Index Array(array=w432, index=w431) -> (element=w433:dbl)
            n185 = Array Subset(array=w432, index=w431) -> (w430:dbl[])  [unwired: 1 in]
            n186 = Add Array Elements(numeric array=w430) -> (sum=w429:dbl)
            n187 = Unbundle By Name(w428) -> ("Step"=w427:i32)
          }
          frame True {
            w439 = 0.0
          }
        }
        n188 = Bundle By Name(cluster=w426, "Current Process"=w410, "Current Fluidic Process"=w420, "Duration(s)"=w408, "Total Duration(s)"=w407) -> (w425:T3)
        n189 = call "Enqueue.vi"("Error In"=w418, "State"=w416, "Queue in"=w417) -> ("Error Out"=w414:errorcluster)  [unwired: 7 in, 1 out]
        n190 = call "SEQ Preview Queue.vi"("error in"=w414) -> ("error out"=w415:errorcluster, "SEQ Data"=w412:T7)  [unwired: 9 in]
        n191 = Bundle By Name(cluster=w412, "Current Process"=w406) -> (w411:T7)
        n192 = call "SEQ Lossy Queue.vi"("error in"=w415, "SEQ Data"=w411) -> ("error out"=w413:errorcluster)  [unwired: 9 in]
      }
      frame "Process End" {
        n193 = call "SEQ Preview Queue.vi"("error in"=w449) -> ("error out"=w448:errorcluster, "SEQ Data"=w446:T7)  [unwired: 9 in]
        n194 = Bundle By Name(cluster=w446, "Fluidic Process Done?"=TRUE) -> (w445:T7)
        n195 = call "SEQ Lossy Queue.vi"("error in"=w448, "SEQ Data"=w445) -> ("error out"=w447:errorcluster)  [unwired: 9 in]
      }
      frame "Syringe Pump Off" {
        n196 = call "Enqueue.vi"("Error In"=w456, "State"="I/O Reset", "Queue in"=w455) -> ("Error Out"=w453:errorcluster)  [unwired: 7 in, 1 out]
        n197 = call "Stop.vi"("Error In"=w453) -> ("Error Out"=w452:errorcluster)  [unwired: 10 in]
        n198 = flat-sequence {
          tunnel: w452 -> [w459]
          tunnel: [w459] -> w451
          frame #0 {
            n199 = Wait (ms)(milliseconds to wait=u32 1000) -> ()  [unwired: 1 out]
          }
        }
      }
      frame "I/O Reset" {
        n200 = call "Enqueue.vi"("Error In"=w465, "State"="Process End", "Queue in"=w464) -> ("Error Out"=w462:errorcluster)  [unwired: 7 in, 1 out]
        n201 = call "Update.vi"("Error In"=w462, "I/O Control"=T6 {"Regulator"={"BL2 (V)"=0.0, "BL1 (V)"=0.0, "BR1 (V)"=0.0, "BR2 (V)"=0.0}, "Buffer Pinch Valve"={"Buffer Load L"=FALSE, "Buffer Load R"=FALSE, "Buffer Chip L"=FALSE, "Buffer Chip R"=FALSE, "Sorting Waste"=FALSE, "Filter Waste"=FALSE, "Reagent Waste"=FALSE, "Buffer Waste"=FALSE, "Wash/Buffer Tank"=TRUE}, "Blood Pinch Valve"={"Load S1"=FALSE, "Load S2"=FALSE, "Blood in"=FALSE}, "Fast Valve"={"Fast Valve 1"=FALSE, "Fast Valve 2"=FALSE}, "Blood Sensor"={"Calibrate Sensor 1"=FALSE, "Calibrate Sensor 2"=FALSE}, "Air Pressure"={"Air Compressor"=FALSE, "Air Compressor Manual"=FALSE}, "Blood Tube Latch1"=FALSE, "Air Valve"=FALSE, "Buffer Pump"=FALSE, "Mirror Change"=enum."Camera Side"}) -> ("Error Out"=w461:errorcluster)  [unwired: 9 in]
      }
      frame "------Error Handler------" {
      }
      frame "Error" {
        n202 = Variant To Data(error in=w472, type=errorcluster {"status"=FALSE, "code"=0, "source"=""} ("error constant"), Variant=w471) -> (data=w473:errorcluster)  [unwired: 1 out]
        n203 = call <vilib>:"Simple Error Handler.vi"("error in (no error)"=w473) -> ()  [unwired: 4 in, 5 out]
      }
      frame "------Close------" {
      }
      frame "Close" {
        n204 = for {
          tunnel: w479 -> [w483]
          shift-right: [w484] -> w478
          shift-left: w480 -> [w485]
          tunnel: string[] ["Release Queue"] -> [w482] mode=indexing
          n205 = call "Enqueue.vi"("Error In"=w485, "State"=w482, "Queue in"=w483) -> ("Error Out"=w484:errorcluster)  [unwired: 7 in, 1 out]
        }
      }
      frame "Release Queue" {
        n206 = Release Queue(queue=w489, error in (no error)=w490) -> (error out=w487:errorcluster)  [unwired: 1 in, 2 out]
        n207 = call "SEQ Release Queue.vi"("error in"=w487) -> ("error out"=w486:errorcluster)  [unwired: 10 in]
      }
    }
    n208 = case shown="Error .." w87 {
      selector: w87 -> [w492 w496]
      tunnel: [w492 w497] -> w88
      tunnel: w86 -> [_ w494]
      frame No Error {
      }
      frame Error {
        n209 = To Variant(anything=w496) -> (Variant=w495:variant)
        n210 = call "Enqueue.vi"("Data"=w495, "State"="Error", "Queue in"=w494) -> ("Error Out"=w497:errorcluster)  [unwired: 7 in, 1 out]
      }
    }
  }
  n211 = Merge Errors(w8, w6) -> (→"error out":errorcluster)
